vi "Bubble_test.vi"(2 "Body Bubble Rad":dbl, 3 "Body Centroid":dbl[](array[numeric]), 4 "Dynamic Facets":T1, 5 "Static Facets":T1) -> (0 "Dynamic working Facet index":i32[](array[numeric]), 1 "Static working Facet index":i32[](array[numeric]))   [LabVIEW 2011]
uses:
  Facet_Array.ctl
  <vilib>/Analysis/baseanly.llb/Unit Vector (DBL).vi
  <vilib>/Analysis/NI_AALBase.lvlib
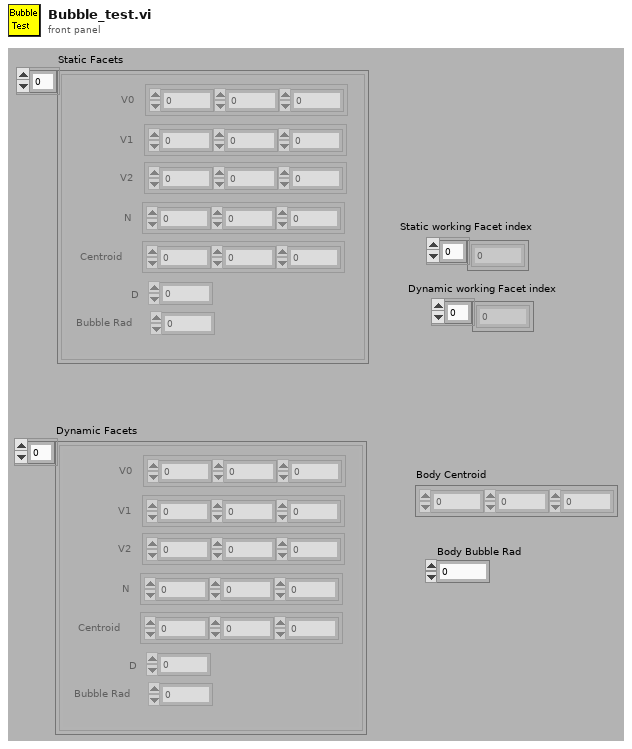
[diagram p1: front panel]
types:
  T1 = typedef "Facet_Array.ctl" = cluster{"V0":dbl[], "V1":dbl[], "V2":dbl[], "N":dbl[], "Centroid":dbl[], "D":dbl, "Bubble Rad":dbl}[]
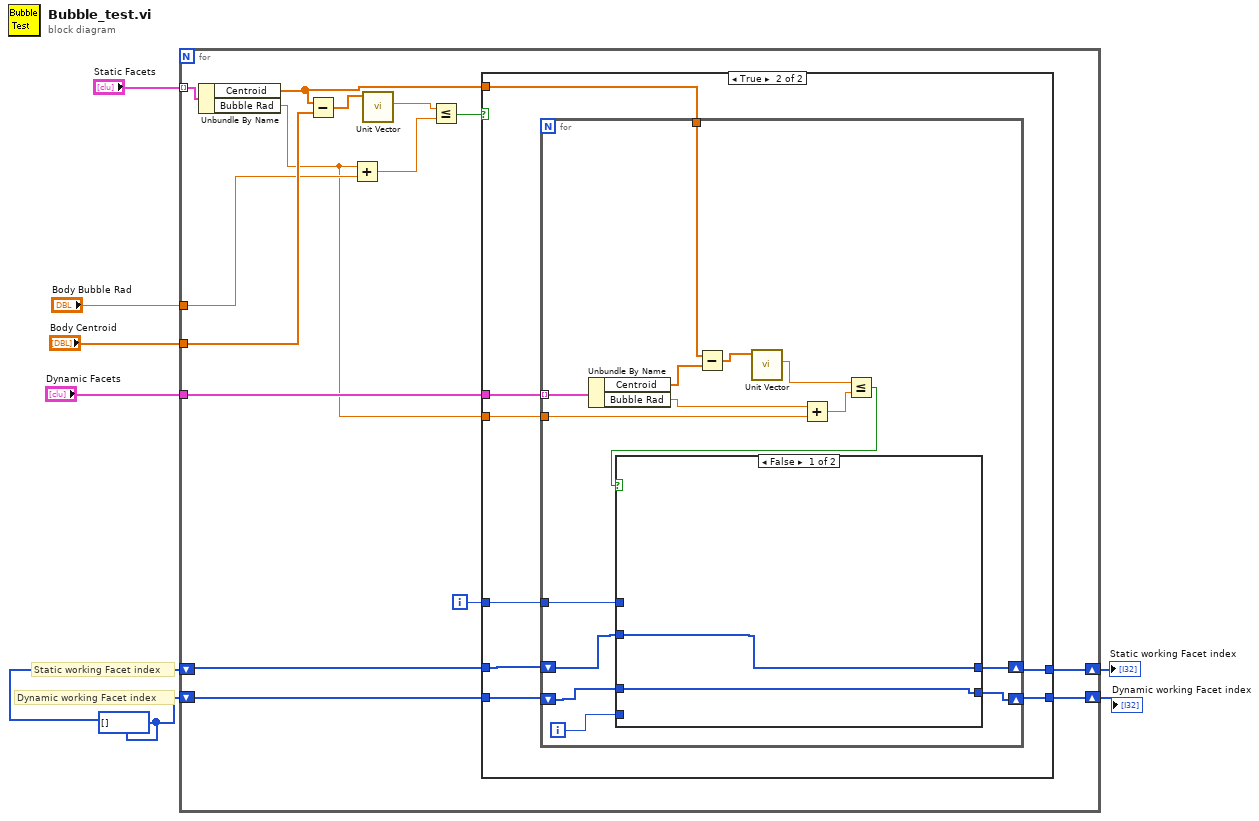
[diagram p0: block diagram]
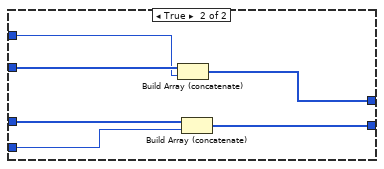
[diagram p3: hidden frame]
diagram:
  w3 = i32[] []
  # "Dynamic working Facet index"
  # "Static working Facet index"
  n1 = for {
    tunnel: "Static Facets" -> [w22] mode=indexing
    tunnel: "Body Centroid" -> [w21]
    tunnel: "Body Bubble Rad" -> [w19]
    shift-right: [w13] -> w1
    shift-left: w3 -> [w12]
    shift-right: [w14] -> w2
    shift-left: w3 -> [w15]
    tunnel: "Dynamic Facets" -> [w11]
    i -> [w8]
    n2 = Unbundle By Name(w22) -> ("Centroid"=w10:dbl[], "Bubble Rad"=w9:dbl)
    n3 = Subtract(x=w10, y=w21) -> (x-y=w20:dbl[])
    n4 = Add(x=w9, y=w19) -> (x+y=w17:dbl)
    n5 = call-poly <vilib>:"Unit Vector.vi"("Input Vector"=w20) -> ("norm"=w18:dbl)  [unwired: 8 in, 2 out]
    n6 = Less Or Equal?(x=w18, y=w17) -> (x <= y?=w16:bool)
    n7 = case shown="True" w16 {
      tunnel: w15 -> [w24 w28]
      tunnel: [w24 w26] -> w14
      tunnel: [w23 w25] -> w13
      tunnel: w12 -> [w23 w27]
      tunnel: w11 -> [_ w32]
      tunnel: w10 -> [_ w31]
      tunnel: w9 -> [_ w30]
      tunnel: w8 -> [_ w29]
      frame False {
      }
      frame True {
        n8 = for {
          tunnel: w32 -> [w47] mode=indexing
          tunnel: w31 -> [w46]
          tunnel: w30 -> [w42]
          tunnel: w29 -> [w38]
          shift-right: [w36] -> w26
          shift-left: w28 -> [w37]
          shift-right: [w33] -> w25
          shift-left: w27 -> [w35]
          i -> [w34]
          n9 = Unbundle By Name(w47) -> ("Centroid"=w45:dbl[], "Bubble Rad"=w43:dbl)
          n10 = Subtract(x=w46, y=w45) -> (x-y=w44:dbl[])
          n11 = call-poly <vilib>:"Unit Vector.vi"("Input Vector"=w44) -> ("norm"=w41:dbl)  [unwired: 8 in, 2 out]
          n12 = Add(x=w43, y=w42) -> (x+y=w40:dbl)
          n13 = Less Or Equal?(x=w41, y=w40) -> (x <= y?=w39:bool)
          n14 = case shown="False" w39 {
            tunnel: w37 -> [w49 w55]
            tunnel: w38 -> [_ w54]
            tunnel: [w49 w53] -> w36
            tunnel: w35 -> [w48 w52]
            tunnel: w34 -> [_ w51]
            tunnel: [w48 w50] -> w33
            frame False {
            }
            frame True {
              n15 = Build Array (concatenate)(w55, w54) -> (w53:i32[])
              n16 = Build Array (concatenate)(w52, w51) -> (w50:i32[])
            }
          }
        }
      }
    }
  }
  "Static working Facet index" <- w2
  "Dynamic working Facet index" <- w1
